vi "Initialize.vi"(8 "Error In":errorcluster, 11 "VI Ref In":refnum<vi>) -> (0 "Error Out":errorcluster, 1 "Executable Configuration":T2, 2 "Data Structures":T1, 3 "Action Queues":T3)   [LabVIEW 2013]
uses:
  ActionQueues.ctl
  UIActionQueueElement.ctl
  UIAction.ctl
  HardwareActionQueueElement.ctl
  HardwareAction.ctl
  LogActionQueueElement.ctl
  LogAction.ctl
  ExecutableConfiguration.ctl
  DataStructures.ctl
  HardwareDisplayData.ctl
  HardwareLogData.ctl
  libs/LV-Utilities/LV-Utilities.lvlib
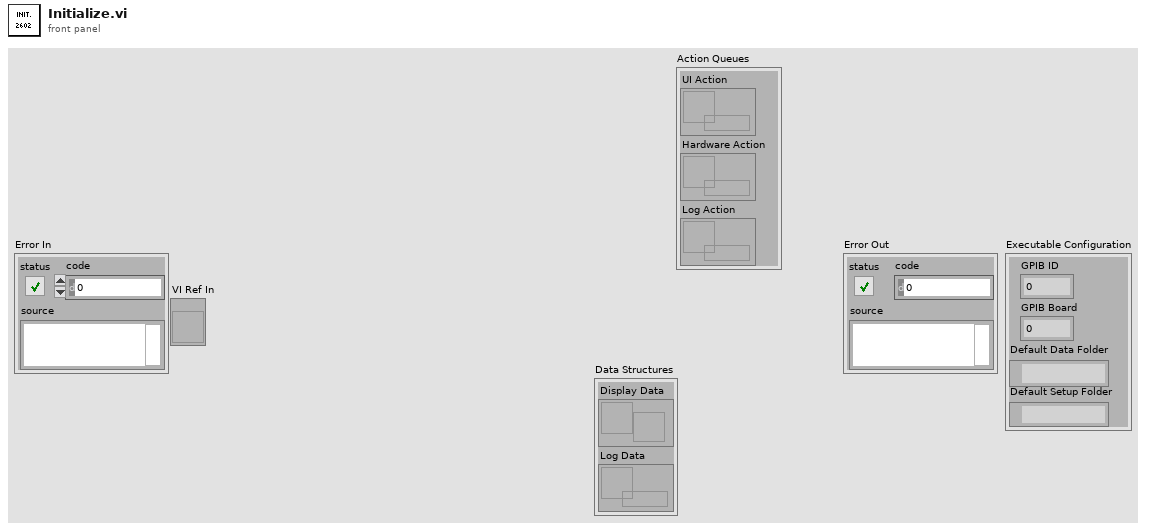
[diagram p1: front panel]
types:
  T1 = typedef "DataStructures.ctl" = cluster{"Display Data":refnum<notifier>, "Log Data":refnum<queue>}
  T2 = typedef "ExecutableConfiguration.ctl" = cluster{"GPIB ID":u8, "GPIB Board":u8, "Default Data Folder":path, "Default Setup Folder":path}
  T3 = typedef "ActionQueues.ctl" = cluster{"UI Action":refnum<queue>, "Hardware Action":refnum<queue>, "Log Action":refnum<queue>}
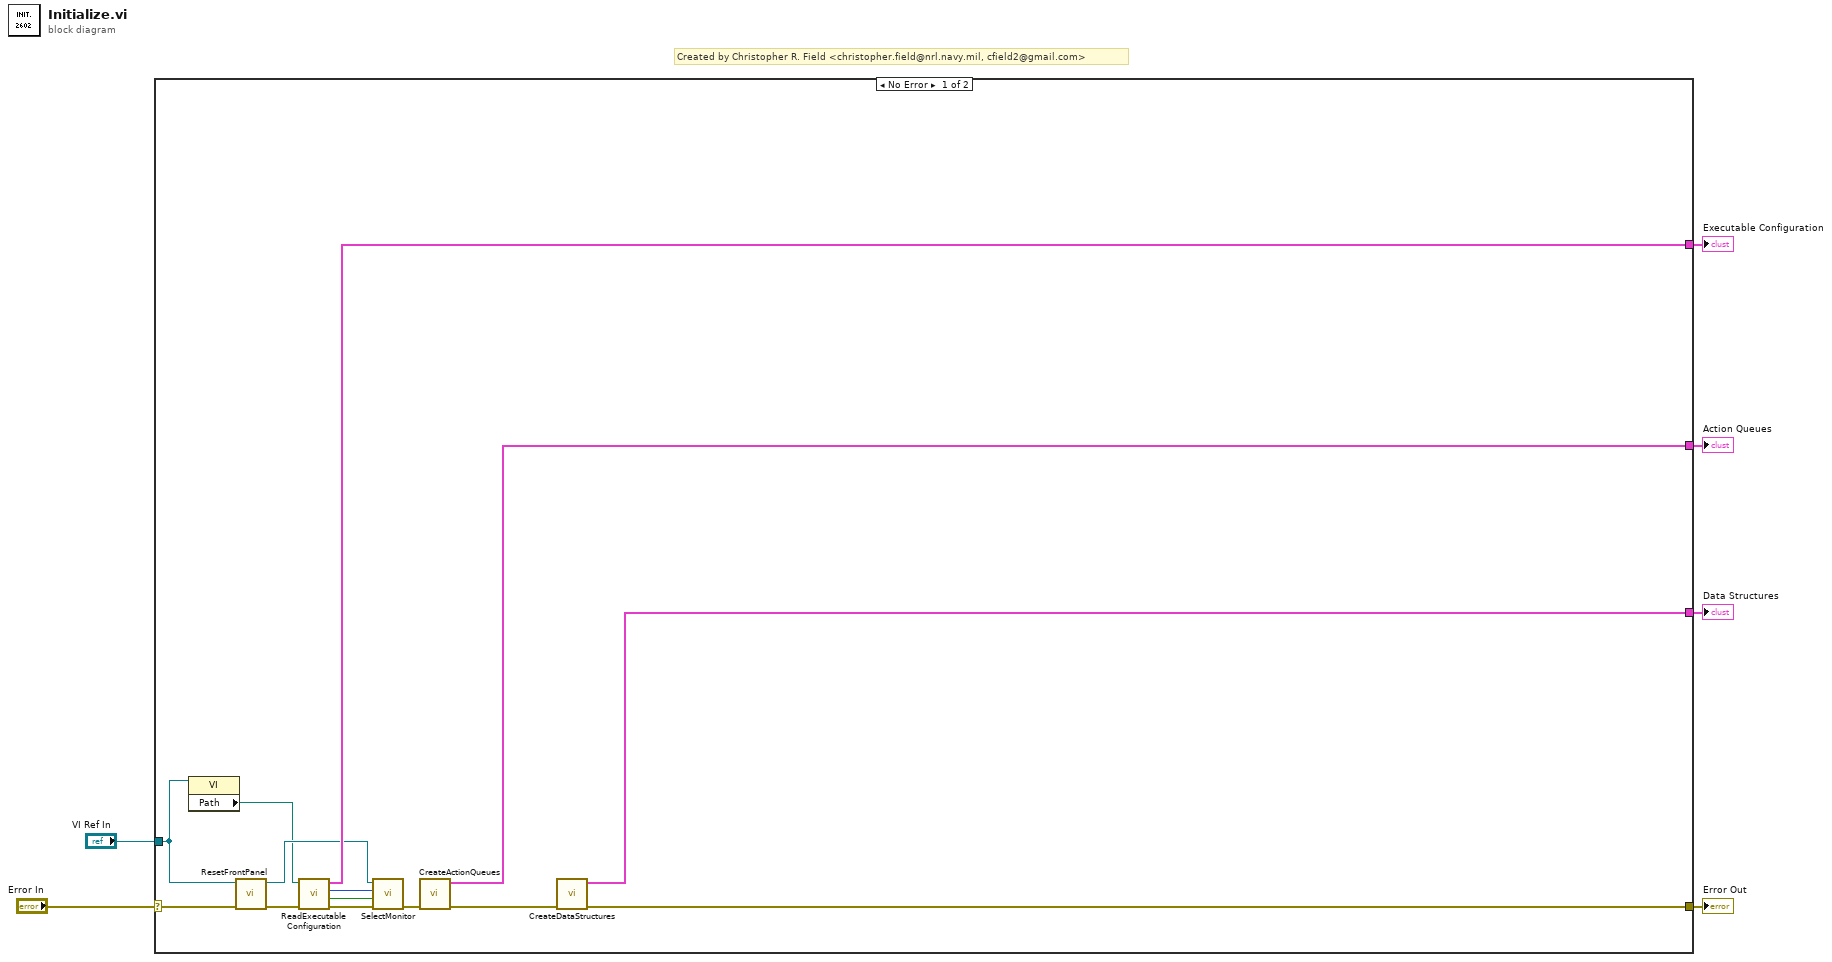
[diagram p0: block diagram]
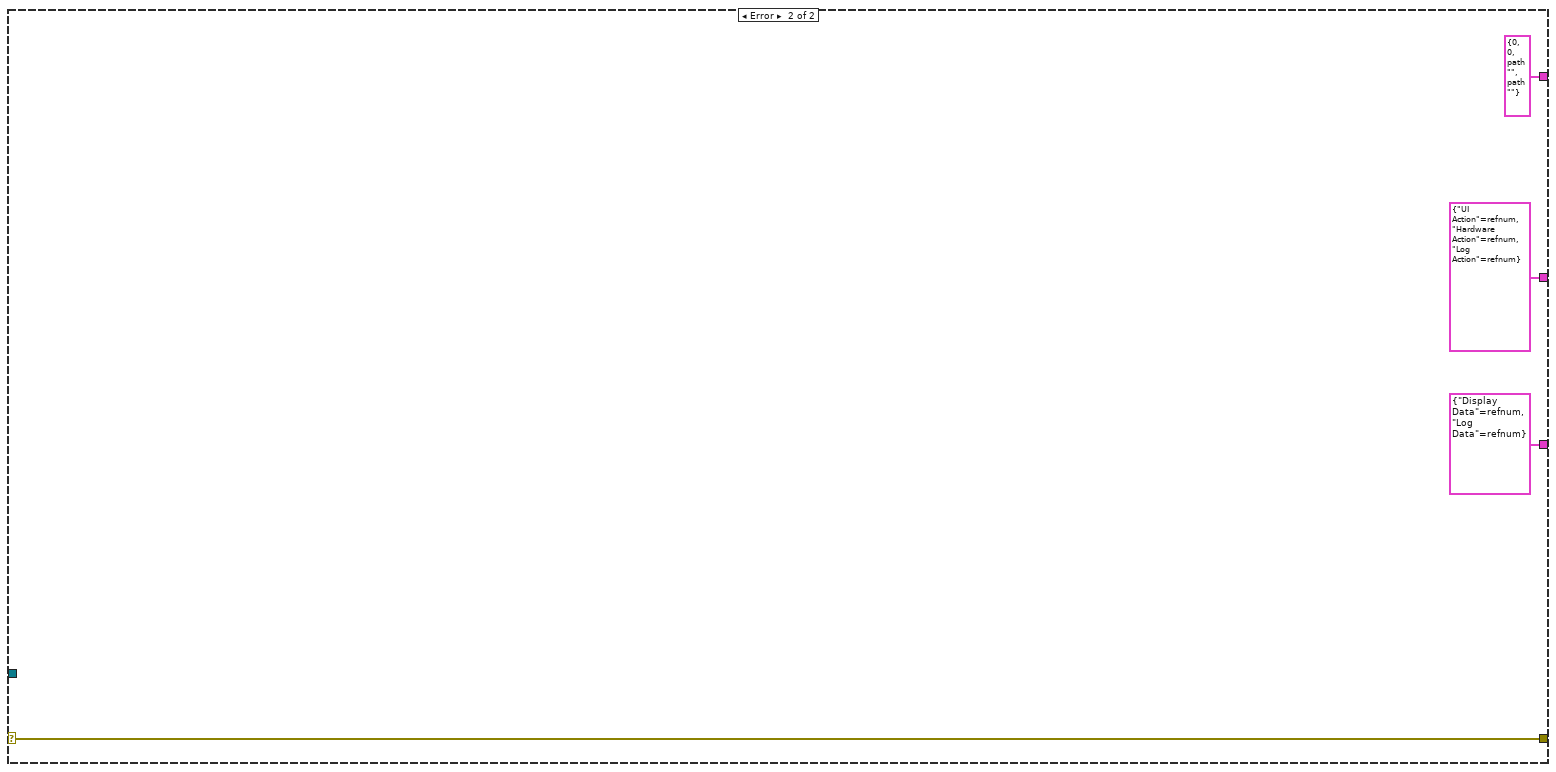
[diagram p2: hidden frame]
diagram:
  # "Created by Christopher R. Field <christopher.field@nrl.navy.mil, cfield2@gmail.com>"
  n1 = case shown="No Error" "Error In" {
    selector: "Error In" -> [w20 w24]
    tunnel: [w13 w24] -> w5
    tunnel: [w18 T3 {"UI Action"=refnum, "Hardware Action"=refnum, "Log Action"=refnum} ("Action Queues")] -> w4
    tunnel: [w16 T2 {"GPIB ID"=0, "GPIB Board"=0, "Default Data Folder"=path "", "Default Setup Folder"=path ""} ("Executable Configuration")] -> w3
    tunnel: [w12 T1 {"Display Data"=refnum, "Log Data"=refnum} ("Data Structures")] -> w2
    tunnel: "VI Ref In" -> [w8 _]
    frame No Error {
      n2 = property class="VI"(reference=w8) -> ("Path"=w7:path)  [unwired: 1 in, 2 out]
      n3 = call "ResetFrontPanel.vi"("Error In"=w20, "VI Ref In"=w8) -> ("Error Out"=w17:errorcluster, "VI Ref Out"=w9:refnum<vi>)  [unwired: 8 in]
      n4 = call "ReadExecutableConfiguration.vi"("Error In"=w17, "VI Path"=w7) -> ("Error Out"=w15:errorcluster, "Center on Monitor?"=w10:bool, "Default Monitor"=w11:i32, "Executable Configuration"=w16:T2)  [unwired: 6 in]
      n5 = call "SelectMonitor.vi"("Error In"=w15, "Center?"=w10, "Monitor (0=primary)"=w11, "VI Ref In"=w9) -> ("Error out"=w19:errorcluster)  [unwired: 6 in, 1 out]
      n6 = call "CreateActionQueues.vi"("Error In"=w19) -> ("Error Out"=w14:errorcluster, "Action Queues"=w18:T3)  [unwired: 9 in]
      n7 = call "CreateDataStructures.vi"("Error In"=w14) -> ("Error Out"=w13:errorcluster, "Data Structures"=w12:T1)  [unwired: 9 in]
    }
    frame Error {
    }
  }
  "Error Out" <- w5
  "Action Queues" <- w4
  "Executable Configuration" <- w3
  "Data Structures" <- w2
